vi "HXG2_GetAllNamesTDMS.vi"(0 "Air-Liq Cluster":T3 {"Liq Cluster"."Liq TEMP %" min=0.0 max=100.0 step=1.0 format="%#.1f"; "Liq Cluster"."Liq FLOW %" min=0.0 max=100.0 step=1.0 format="%#.1f"; "Liq Cluster"."TLiq °F" min=40.0 max=180.0 step=1.0 format="%#.1f"; "Liq Cluster"."Mdot lbm/hr" min=0.0 max=1000.0 step=1.0 format="%#.1f"; "Air Cluster"."Air TEMP %" min=0.0 max=100.0 step=1.0 format="%#.1f"; "Air Cluster"."Air FLOW %" min=0.0 max=100.0 step=1.0 format="%#.1f"; "Air Cluster"."Tair  °F" min=-5.0 max=100.0 step=1.0 format="%#.1f"; "Air Cluster"."CFMs" min=0.0 max=200.0 step=1.0 format="%#.1f"}, 1 "Calcs":T6, 2 "DATA In":T7, 3 "Test Point":i32, 4 "Excel/Elapsed t":dbl[](array[numeric]), 5 "error in (no error)":errorcluster, 6 "Control":enum16{"Initialize", "Pass"}(ring)) -> (7 "SetPoints":dbl[][](array[numeric]), 10 "Cluster":T1, 11 "Other Data":dbl[][](array[numeric]), 12 "For CoilDesigner":T2[][](array[typedef]) format="%#.1f", 13 "All Temps":dbl[][](array[numeric]), 14 "Means":dbl[][](array[numeric]), 15 "Air Props":dbl[][](array[numeric]), 17 "Liq Props":dbl[][](array[numeric]), 18 "Syst Data":dbl[][](array[numeric]), 19 "error out":errorcluster)   [LabVIEW 2012]
uses:
  Controls/HXG2_AnalogIn.ctl
  Controls/HXG2_Calculated.ctl
  Controls/HXG2_AirGly-Cluster.ctl
  Controls/UI/HXG2_UI_ControlSetAir.ctl
  Controls/UI/HXG2_UI_ControlSetGly.ctl
  Controls/UI/HXG2_NumDisplayLarge.ctl
  PID/HXG2pid.ctl
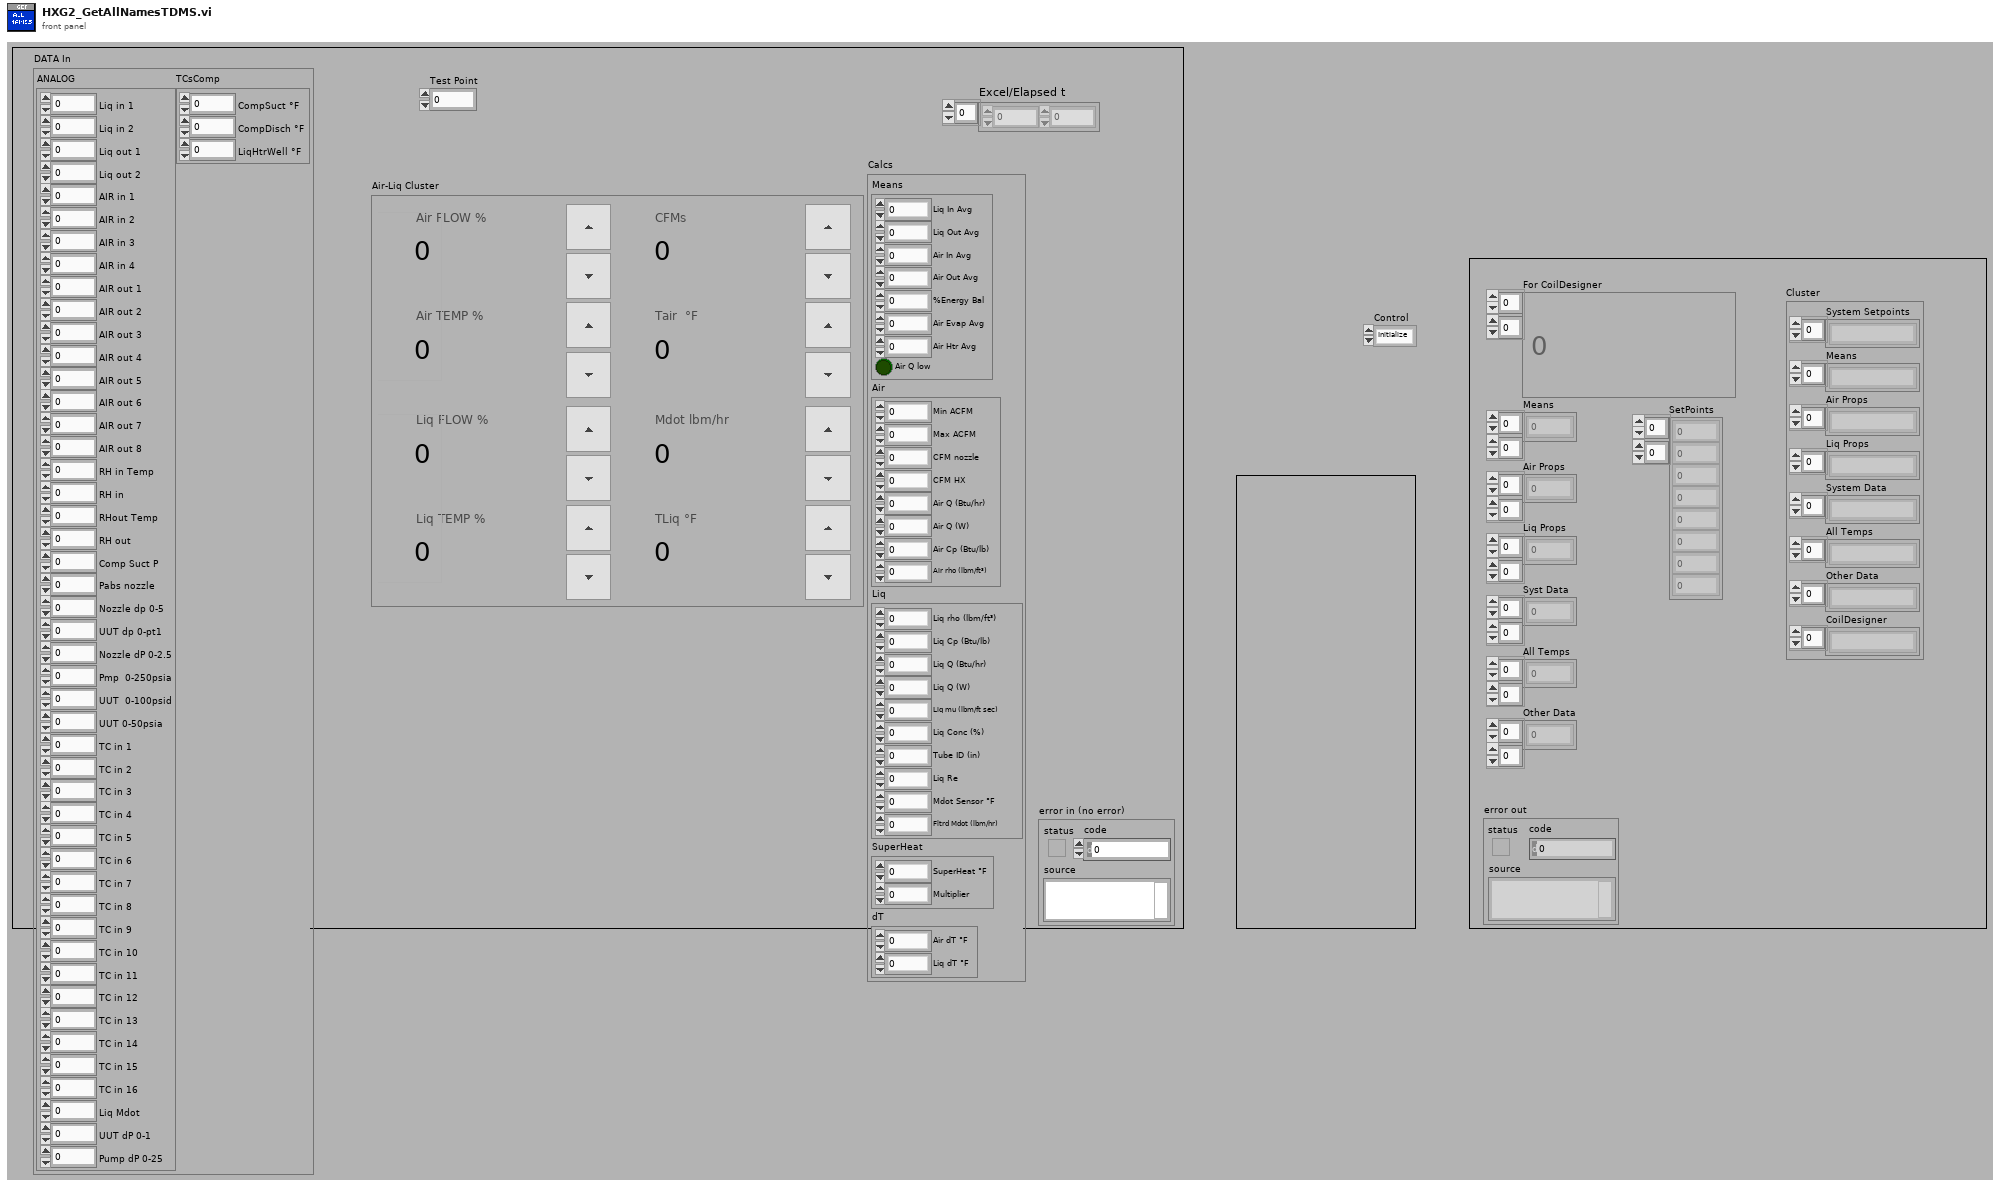
[diagram p1: front panel]
types:
  T1 = cluster{"System Setpoints":string[], "Means":string[], "Air Props":string[], "Liq Props":string[], "System Data":string[], "All Temps":string[], "Other Data":string[], "CoilDesigner":string[]}
  T2 = typedef "HXG2_NumDisplayLarge.ctl" = dbl
  T3 = typedef "HXG2_AirGly-Cluster.ctl" = cluster{"Air Cluster":T4, "Liq Cluster":T5}
  T4 = typedef "HXG2_UI_ControlSetAir.ctl" = cluster{"Air FLOW %":dbl, "Air TEMP % ":dbl, "CFMs":dbl, "Tair  °F":dbl}
  T5 = typedef "HXG2_UI_ControlSetGly.ctl" = cluster{"Liq FLOW %":dbl, "Liq TEMP % ":dbl, "Mdot lbm/hr":dbl, "TLiq °F":dbl}
  T6 = typedef "HXG2_Calculated.ctl" = cluster{"Means":cluster{"Liq In Avg":dbl, "Liq Out Avg":dbl, "Air In Avg":dbl, "Air Out Avg":dbl, "%Energy Bal":dbl, "Air Evap Avg":dbl, "Air Htr Avg":dbl, "Air Q low":bool}, "Air":cluster{"Min ACFM":dbl, "Max ACFM":dbl, "CFM nozzle":dbl, "CFM HX":dbl, "Air Q (Btu/hr)":dbl, "Air Q (W)":dbl, "Air Cp (Btu/lb)":dbl, "Air rho (lbm/ft³)":dbl}, "Liq":cluster{"Liq rho (lbm/ft³)":dbl, "Liq Cp (Btu/lb)":dbl, "Liq Q (Btu/hr)":dbl, "Liq Q (W)":dbl, "Liq mu (lbm/ft sec)":dbl, "Liq Conc (%)":dbl, "Tube ID (in)":dbl, "Liq Re":dbl, "Mdot Sensor °F":dbl, "Fltrd Mdot (lbm/hr)":dbl}, "SuperHeat":cluster{"SuperHeat °F":dbl, "Multiplier":dbl}, "dT":cluster{"Air dT °F":dbl, "Liq dT °F":dbl}}
  T7 = typedef "HXG2_AnalogIn.ctl" = cluster{"ANALOG":cluster{"Liq in 1":dbl, "Liq in 2":dbl, "Liq out 1":dbl, "Liq out 2":dbl, "AIR in 1":dbl, "AIR in 2":dbl, "AIR in 3":dbl, "AIR in 4":dbl, "AIR out 1":dbl, "AIR out 2":dbl, "AIR out 3":dbl, "AIR out 4":dbl, "AIR out 5":dbl, "AIR out 6":dbl, "AIR out 7":dbl, "AIR out 8":dbl, "RH in Temp":dbl, "RH in":dbl, "RHout Temp":dbl, "RH out":dbl, "Comp Suct P":dbl, "Pabs nozzle":dbl, "Nozzle dp 0-5":dbl, "UUT dp 0-pt1":dbl, "Nozzle dP 0-2.5":dbl, "Pmp  0-250psia":dbl, "UUT  0-100psid":dbl, "UUT 0-50psia":dbl, "TC in 1":dbl, "TC in 2":dbl, "TC in 3":dbl, "TC in 4":dbl, "TC in 5":dbl, "TC in 6":dbl, "TC in 7":dbl, "TC in 8":dbl, "TC in 9":dbl, "TC in 10":dbl, "TC in 11":dbl, "TC in 12":dbl, "TC in 13":dbl, "TC in 14":dbl, "TC in 15":dbl, "TC in 16":dbl, "Liq Mdot":dbl, "UUT dP 0-1":dbl, "Pump dP 0-25":dbl}, "TCsComp":cluster{"CompSuct °F  ":dbl, "CompDisch °F":dbl, "LiqHtrWell °F":dbl}}
  T8 = typedef "HXG2pid.ctl" = enum16{"Write PID Efforts", "Write PID On-Off", "Pass", "Write PID Refs", "Write PID Gains", "Wrt PID Resets"}
  T9 = cluster{"Excel/Elapsed t[0]":dbl, "Excel/Elapsed t[1]":dbl}
  T10 = cluster{"Liq in 1":dbl, "Liq in 2":dbl, "Liq out 1":dbl, "Liq out 2":dbl, "AIR in 1":dbl, "AIR in 2":dbl, "AIR in 3":dbl, "AIR in 4":dbl, "AIR out 1":dbl, "AIR out 2":dbl, "AIR out 3":dbl, "AIR out 4":dbl, "AIR out 5":dbl, "AIR out 6":dbl, "AIR out 7":dbl, "AIR out 8":dbl, "RH in Temp":dbl, "RH in":dbl, "RHout Temp":dbl, "RH out":dbl, "Comp Suct P":dbl, "Pabs nozzle":dbl, "Nozzle dp 0-5":dbl, "UUT dp 0-pt1":dbl, "Nozzle dP 0-2.5":dbl, "Pmp  0-250psia":dbl, "UUT  0-100psid":dbl, "UUT 0-50psia":dbl, "TC in 1":dbl, "TC in 2":dbl, "TC in 3":dbl, "TC in 4":dbl, "TC in 5":dbl, "TC in 6":dbl, "TC in 7":dbl, "TC in 8":dbl, "TC in 9":dbl, "TC in 10":dbl, "TC in 11":dbl, "TC in 12":dbl, "TC in 13":dbl, "TC in 14":dbl, "TC in 15":dbl, "TC in 16":dbl, "Liq Mdot":dbl, "UUT dP 0-1":dbl, "Pump dP 0-25":dbl}
  T11 = typedef "HXG2_PIDctrlsOUT.ctl" = cluster{"Iteration dT (s)":dbl, "af ctrl effort":dbl, "ac ctrl effort":dbl, "ah ctrl effort":dbl, "lf ctrl effort":dbl, "lc ctrl effort":dbl, "lh ctrl effort":dbl}
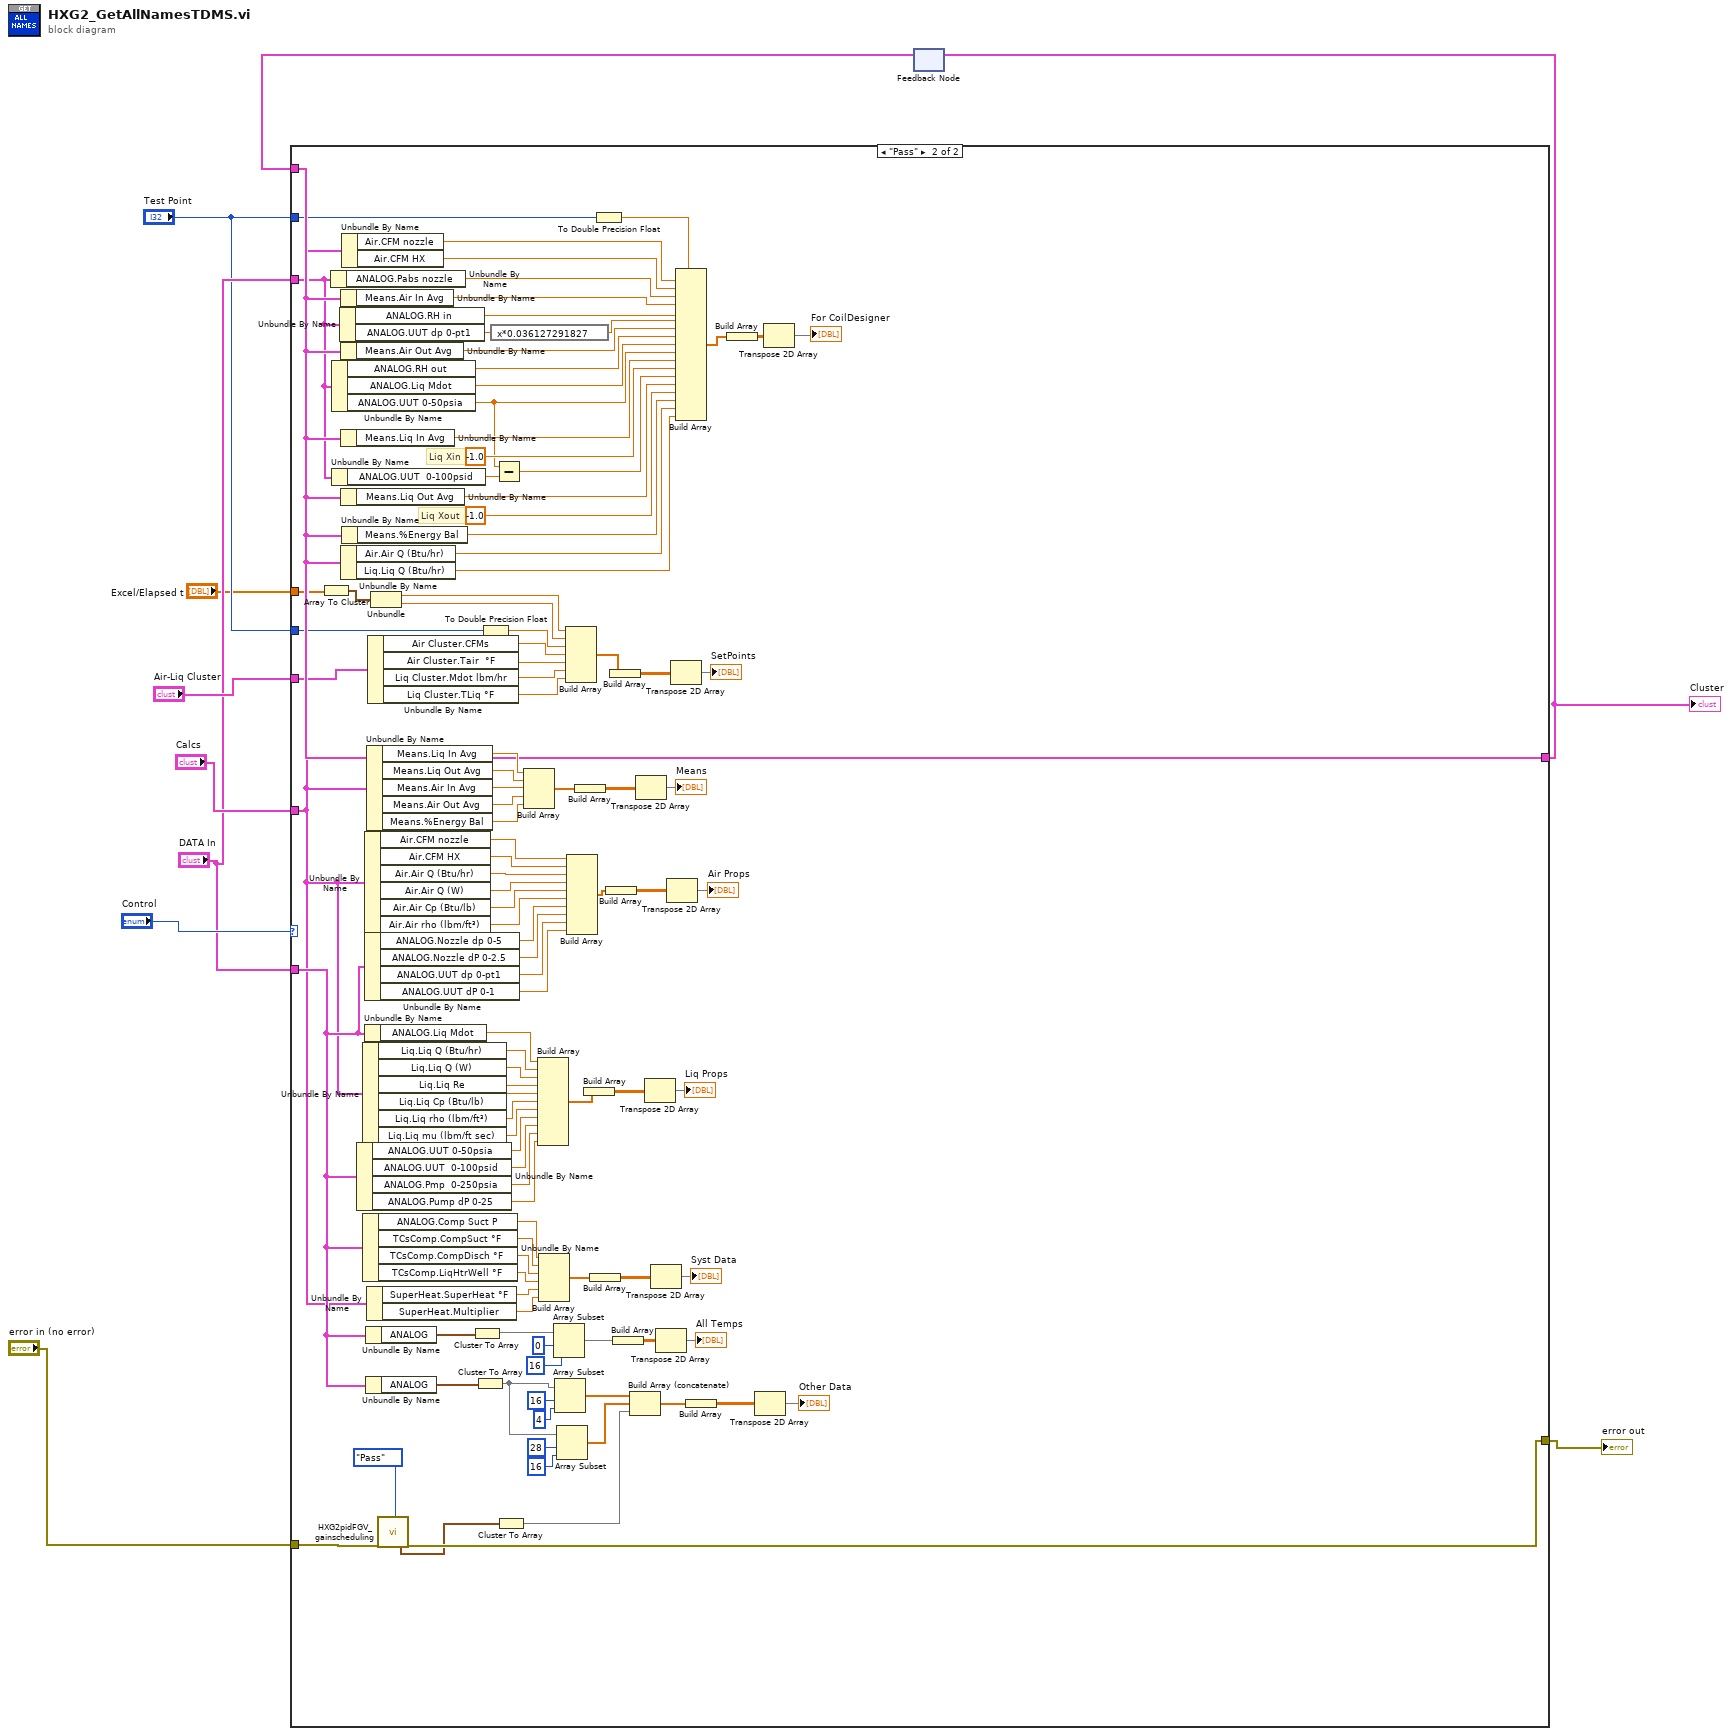
[diagram p0: block diagram]
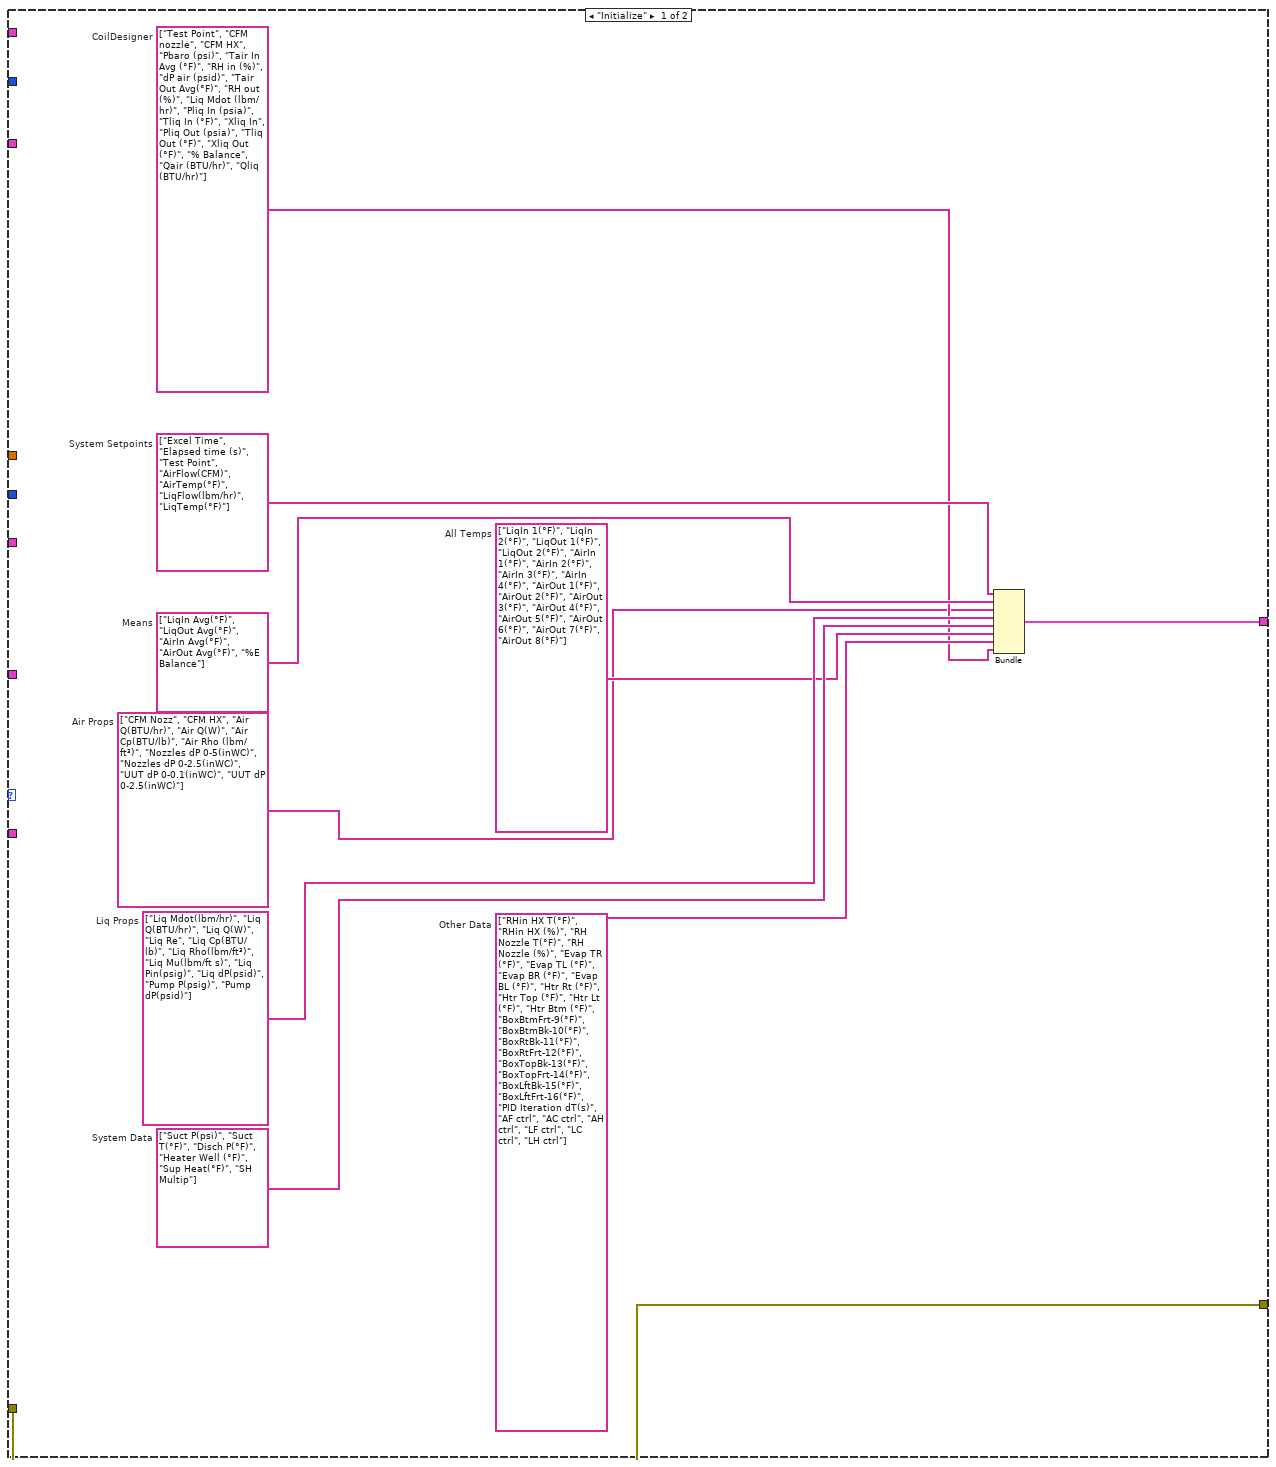
[diagram p2: hidden frame]
diagram:
  n1 = feedback #1() -> (w5:T1)  [unwired: 1 in]
  n2 = case shown="\"Pass\"" "Control" {
    tunnel: [w13 w75] -> w6
    tunnel: "Air-Liq Cluster" -> [_ w54]
    tunnel: "Calcs" -> [_ w39]
    tunnel: "DATA In" -> [_ w96]
    tunnel: "error in (no error)" -> [w20 w24]
    tunnel: [w20 w23] -> w7
    tunnel: w5 -> [_ w75]
    tunnel: "DATA In" -> [_ w28]
    tunnel: "Test Point" -> [_ w44]
    tunnel: "Test Point" -> [_ w43]
    tunnel: "Excel/Elapsed t" -> [_ w36]
    frame "Initialize" {
      w11 = string[] ["CFM Nozz", "CFM HX", "Air Q(BTU/hr)", "Air Q(W)", "Air Cp(BTU/lb)", "Air Rho (lbm/ft³)", "Nozzles dP 0-5(inWC)", "Nozzles dP 0-2.5(inWC)", "UUT dP 0-0.1(inWC)", "UUT dP 0-2.5(inWC)"]  # Air Props
      w12 = string[] ["Test Point", "CFM nozzle", "CFM HX", "Pbaro (psi)", "Tair In Avg (°F)", "RH in (%)", "dP air (psid)", "Tair Out Avg(°F)", "RH out (%)", "Liq Mdot (lbm/hr)", "Pliq In (psia)", "Tliq In (°F)", "Xliq In", "Pliq Out (psia)", "Tliq Out (°F)", "Xliq Out (°F)", "% Balance", "Qair (BTU/hr)", "Qliq (BTU/hr)"]  # CoilDesigner
      w14 = string[] ["RHin HX T(°F)", "RHin HX (%)", "RH Nozzle T(°F)", "RH Nozzle (%)", "Evap TR (°F)", "Evap TL (°F)", "Evap BR (°F)", "Evap BL (°F)", "Htr Rt (°F)", "Htr Top (°F)", "Htr Lt (°F)", "Htr Btm (°F)", "BoxBtmFrt-9(°F)", "BoxBtmBk-10(°F)", "BoxRtBk-11(°F)", "BoxRtFrt-12(°F)", "BoxTopBk-13(°F)", "BoxTopFrt-14(°F)", "BoxLftBk-15(°F)", "BoxLftFrt-16(°F)", "PID Iteration dT(s)", "AF ctrl", "AC ctrl", "AH ctrl", "LF ctrl", "LC ctrl", "LH ctrl"]  # Other Data
      w15 = string[] ["LiqIn 1(°F)", "LiqIn 2(°F)", "LiqOut 1(°F)", "LiqOut 2(°F)", "AirIn 1(°F)", "AirIn 2(°F)", "AirIn 3(°F)", "AirIn 4(°F)", "AirOut 1(°F)", "AirOut 2(°F)", "AirOut 3(°F)", "AirOut 4(°F)", "AirOut 5(°F)", "AirOut 6(°F)", "AirOut 7(°F)", "AirOut 8(°F)"]  # All Temps
      w16 = string[] ["Suct P(psi)", "Suct T(°F)", "Disch P(°F)", "Heater Well (°F)", "Sup Heat(°F)", "SH Multip"]  # System Data
      w17 = string[] ["Liq Mdot(lbm/hr)", "Liq Q(BTU/hr)", "Liq Q(W)", "Liq Re", "Liq Cp(BTU/lb)", "Liq Rho(lbm/ft³)", "Liq Mu(lbm/ft s)", "Liq Pin(psig)", "Liq dP(psid)", "Pump P(psig)", "Pump dP(psid)"]  # Liq Props
      w18 = string[] ["LiqIn Avg(°F)", "LiqOut Avg(°F)", "AirIn Avg(°F)", "AirOut Avg(°F)", "%E Balance"]  # Means
      w19 = string[] ["Excel Time", "Elapsed time (s)", "Test Point", "AirFlow(CFM)", "AirTemp(°F)", "LiqFlow(lbm/hr)", "LiqTemp(°F)"]  # System Setpoints
      n3 = Bundle("System Setpoints"=w19, "Means"=w18, "Air Props"=w11, "Liq Props"=w17, "System Data"=w16, "All Temps"=w15, "Other Data"=w14, "CoilDesigner"=w12) -> (w13:T1)  [unwired: 1 in]
    }
    frame "Pass" {
      # "Liq Xout"
      # "Liq Xin"
      n4 = Array To Cluster(array=w36) -> (cluster=w35:T9)
      n5 = Unbundle By Name(w28) -> ("ANALOG.Pabs nozzle"=w27:dbl)
      n6 = Unbundle By Name(w28) -> ("ANALOG.RH out"=w62:dbl, "ANALOG.Liq Mdot"=w45:dbl, "ANALOG.UUT 0-50psia"=w26:dbl)
      n7 = Unbundle By Name(w28) -> ("ANALOG.UUT  0-100psid"=w69:dbl)
      n8 = Unbundle By Name(w28) -> ("ANALOG.RH in"=w65:dbl, "ANALOG.UUT dp 0-pt1"=w46:dbl)
      n9 = Unbundle By Name(w39) -> ("Means.Air In Avg"=w66:dbl)
      n10 = Unbundle By Name(w39) -> ("Means.Air Out Avg"=w63:dbl)
      n11 = Unbundle By Name(w39) -> ("Means.Liq In Avg"=w61:dbl)
      n12 = Unbundle By Name(w39) -> ("Means.Liq Out Avg"=w58:dbl)
      n13 = Unbundle By Name(w39) -> ("Air.Air Q (Btu/hr)"=w38:dbl, "Liq.Liq Q (Btu/hr)"=w37:dbl)
      n14 = Unbundle By Name(w39) -> ("Air.CFM nozzle"=w68:dbl, "Air.CFM HX"=w67:dbl)
      n15 = Unbundle By Name(w39) -> ("Means.%Energy Bal"=w56:dbl)
      n16 = Unbundle By Name(w96) -> ("ANALOG.UUT 0-50psia"=w101:dbl, "ANALOG.UUT  0-100psid"=w100:dbl, "ANALOG.Pmp  0-250psia"=w31:dbl, "ANALOG.Pump dP 0-25"=w30:dbl)
      n17 = Unbundle By Name(w39) -> ("Liq.Liq Q (Btu/hr)"=w114:dbl, "Liq.Liq Q (W)"=w115:dbl, "Liq.Liq Re"=w116:dbl, "Liq.Liq Cp (Btu/lb)"=w117:dbl, "Liq.Liq rho (lbm/ft³)"=w118:dbl, "Liq.Liq mu (lbm/ft sec)"=w119:dbl)
      n18 = Unbundle By Name(w96) -> ("ANALOG.Comp Suct P"=w112:dbl, "TCsComp.CompSuct °F"=w111:dbl, "TCsComp.CompDisch °F"=w110:dbl, "TCsComp.LiqHtrWell °F"=w29:dbl)
      n19 = Unbundle By Name(w39) -> ("Air.CFM nozzle"=w125:dbl, "Air.CFM HX"=w124:dbl, "Air.Air Q (Btu/hr)"=w123:dbl, "Air.Air Q (W)"=w122:dbl, "Air.Air Cp (Btu/lb)"=w121:dbl, "Air.Air rho (lbm/ft³)"=w120:dbl)
      n20 = Unbundle By Name(w96) -> ("ANALOG.Nozzle dp 0-5"=w103:dbl, "ANALOG.Nozzle dP 0-2.5"=w102:dbl, "ANALOG.UUT dp 0-pt1"=w40:dbl, "ANALOG.UUT dP 0-1"=w32:dbl)
      n21 = Unbundle By Name(w96) -> ("ANALOG.Liq Mdot"=w113:dbl)
      n22 = Unbundle By Name(w96) -> ("ANALOG"=w107:T10)
      n23 = Unbundle By Name(w96) -> ("ANALOG"=w97:T10)
      n24 = Unbundle By Name(w39) -> ("Means.Liq In Avg"=w130:dbl, "Means.Liq Out Avg"=w129:dbl, "Means.Air In Avg"=w128:dbl, "Means.Air Out Avg"=w127:dbl, "Means.%Energy Bal"=w126:dbl)
      n25 = Unbundle By Name(w39) -> ("SuperHeat.SuperHeat °F"=w109:dbl, "SuperHeat.Multiplier"=w108:dbl)
      n26 = Unbundle By Name(w54) -> ("Air Cluster.CFMs"=w53:dbl, "Air Cluster.Tair  °F"=w52:dbl, "Liq Cluster.Mdot lbm/hr"=w51:dbl, "Liq Cluster.TLiq °F"=w50:dbl)
      n27 = Unbundle(w35) -> ("Excel/Elapsed t[0]"=w33:dbl, "Excel/Elapsed t[1]"=w34:dbl)
      n28 = call "HXG2pidFGV_gainscheduling.vi"("error in (no error)"=w24, "PIDfgvCtrl"=HXG2pid."Pass") -> ("PID Ctrls Out"=w22:T11, "error out"=w23:errorcluster)  [unwired: 9 in, 7 out]
      n29 = Cluster To Array(cluster=w107) -> (array=w106:dbl[])
      n30 = Cluster To Array(cluster=w97) -> (array=w71:dbl[])
      n31 = To Double Precision Float(number=w43) -> (double precision float=w41:dbl)
      n32 = expression code="x*0.036127291827"(w46) -> (w64:dbl)
      n33 = Subtract(x=w26, y=w69) -> (x-y=w59:dbl)
      n34 = Cluster To Array(cluster=w22) -> (array=w21:dbl[])
      n35 = Build Array(w130, w129, w128, w127, w126) -> (w92:dbl[])
      n36 = Build Array(w113, w114, w115, w116, w117, w118, w119, w101, w100, w31, w30) -> (w86:dbl[])
      n37 = Build Array(w112, w111, w110, w29, w109, w108) -> (w83:dbl[])
      n38 = Array Subset(array=w106, index=0, length=16 ("index")) -> (w81:dbl[])
      n39 = Array Subset(array=w71, index=16, length=4 ("index")) -> (w72:dbl[])
      n40 = Array Subset(array=w71, index=28, length=16 ("index")) -> (w70:dbl[])
      n41 = Build Array(w33, w34, w41, w53, w52, w51, w50) -> (w47:dbl[])
      n42 = Build Array(w125, w124, w123, w122, w121, w120, w103, w102, w40, w32) -> (w89:dbl[])
      n43 = Build Array(w92) -> (w93:dbl[][])
      n44 = Build Array(w86) -> (w87:dbl[][])
      n45 = Build Array(w83) -> (w84:dbl[][])
      n46 = To Double Precision Float(number=w44) -> (double precision float=w42:dbl)
      n47 = Build Array(w89) -> (w90:dbl[][])
      n48 = Build Array(w47) -> (w48:dbl[][])
      n49 = Build Array(w81) -> (w80:dbl[][])
      n50 = Build Array (concatenate)(w72, w70, w21) -> (w77:dbl[])
      n51 = Transpose 2D Array(2D array=w93) -> (transposed array=→"Means":dbl[][])
      n52 = Transpose 2D Array(2D array=w87) -> (transposed array=→"Liq Props":dbl[][])
      n53 = Transpose 2D Array(2D array=w84) -> (transposed array=→"Syst Data":dbl[][])
      n54 = Transpose 2D Array(2D array=w80) -> (transposed array=→"All Temps":dbl[][])
      n55 = Transpose 2D Array(2D array=w90) -> (transposed array=→"Air Props":dbl[][])
      n56 = Transpose 2D Array(2D array=w48) -> (transposed array=→"SetPoints":dbl[][])
      n57 = Build Array(w42, w68, w67, w27, w66, w65, w64, w63, w62, w45, w26, w61, -1.0, w59, w58, -1.0, w56, w38, w37) -> (w55:dbl[])
      n58 = Build Array(w77) -> (w78:dbl[][])
      n59 = Build Array(w55) -> (w95:dbl[][])
      n60 = Transpose 2D Array(2D array=w78) -> (transposed array=→"Other Data":dbl[][])
      n61 = Transpose 2D Array(2D array=w95) -> (transposed array=→"For CoilDesigner":dbl[][])
    }
  }
  "error out" <- w7
  "Cluster" <- w6
  n62 = feedback-in #1(w6) -> ()
